vi "Configure Output Level.vi"(8 "error in (no error)":errorcluster, 9 "Output Level (0)":dbl, 10 "Output Type (0: Voltage)":u16(ring) items=["Voltage", "Current"], 11 "VISA resource name":refnum<visa-resource-name>) -> (0 "error out":errorcluster, 3 "VISA resource name out":refnum<visa-resource-name>)   [LabVIEW 2013, in "DmmPwr Simulator.lvlib"]
doc: "Configures the current or voltage output."
uses:
  <instrlib>/DmmPwr Simulator/DmmPwr Simulator.lvlib
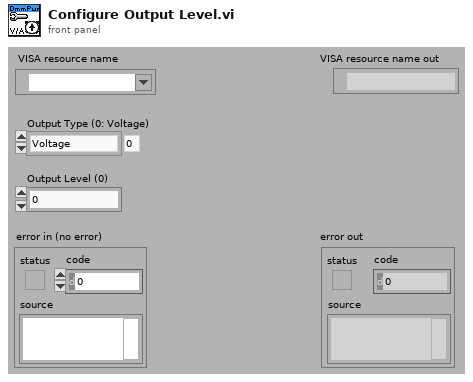
[diagram p1: front panel]
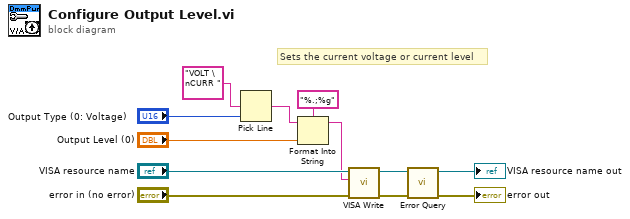
[diagram p0: block diagram]
diagram:
  # "Sets the current voltage or current level"
  n1 = Pick Line(multi-line string="VOLT \nCURR ", line index="Output Type (0: Voltage)") -> (output string=w10:string)  [unwired: 1 in]
  n2 = Format Into String(format string="%.;%g", initial string=w10, "Output Level (0)") -> (resulting string=w1:string)  [unwired: 1 in, 1 out]
  n3 = call <instrlib>:"VISA Write.vi"("error in"="error in (no error)", "write buffer"=w1, "VISA resource name"="VISA resource name") -> ("error out"=w2:errorcluster, "VISA resource name out"=w3:refnum<visa-resource-name>)  [unwired: 6 in, 1 out]
  n4 = call <instrlib>:"Error Query.vi"("error in (no error)"=w2, "VISA resource name"=w3) -> ("error out"=→"error out":errorcluster, "VISA resource name out"=→"VISA resource name out":refnum<visa-resource-name>)  [unwired: 6 in, 2 out]
